vi "Read phone_number.vi"(8 "error in (no error)":errorcluster, 11 "Telegram Class in":refnum<class "Telegram Class.lvclass">) -> (0 "error out":errorcluster, 2 "phone_number":string="7 920-283-83-42", 3 "Telegram Class out":refnum<class "Telegram Class.lvclass">)   [LabVIEW 2015, in "Telegram Library.lvlib" / "Telegram Class.lvclass"]
doc: "Created IvanLis by LabVIEW Portal\nProfile: http://labviewportal.org/memberlist.php?mode=viewprofile&u=987\neMail: IvanLisanov@gMail.com\nTelegram: https://t.me/IvanLis"
uses:
  Telegram Class.lvclass
  Telegram Class.lvclass/Telegram Class.ctl
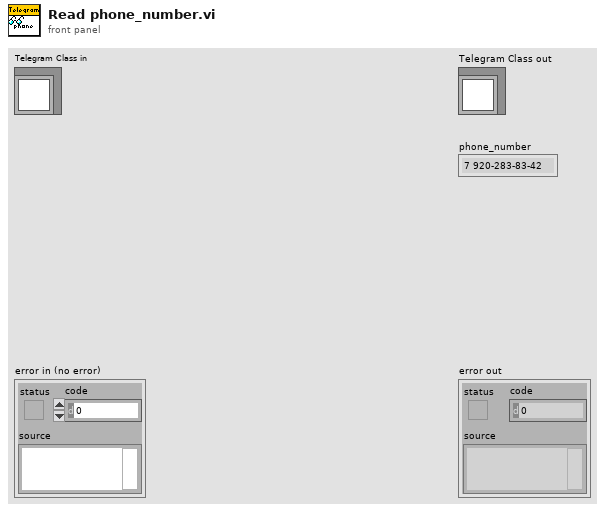
[diagram p1: front panel]
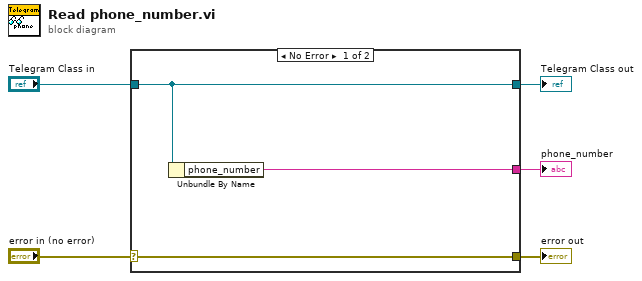
[diagram p0: block diagram]
diagram:
  n1 = case shown="No Error" "error in (no error)" {
    selector: "error in (no error)" -> [w8 w9]
    tunnel: [w8 w9] -> w4
    tunnel: [w7 w10] -> w2
    tunnel: "Telegram Class in" -> [w7 w10]
    tunnel: [w6 _] -> w1
    frame No Error {
      n2 = Unbundle By Name(w7) -> ("phone_number"=w6:string)
    }
    frame Error {
    }
  }
  "error out" <- w4
  "Telegram Class out" <- w2
  "phone_number" <- w1
